vi "Save Shooting Info.vi"(1 "Turret":dbl, 2 "Pitch":dbl, 3 "RPM":dbl) -> ()   [LabVIEW 2011]
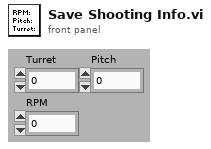
[diagram p1: front panel]
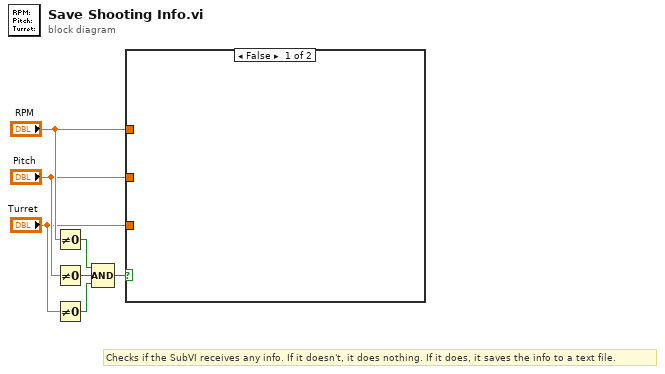
[diagram p0: block diagram]
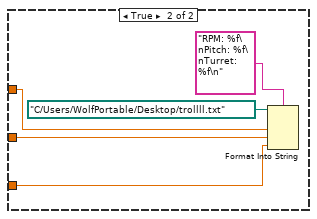
[diagram p2: hidden frame]
diagram:
  # "Checks if the SubVI receives any info. If it doesn't, it does nothing. If it does, it saves the info to a text file."
  n1 = Not Equal To 0?(x="RPM") -> (x != 0?=w7:bool)
  n2 = Not Equal To 0?(x="Pitch") -> (x != 0?=w6:bool)
  n3 = Not Equal To 0?(x="Turret") -> (x != 0?=w5:bool)
  n4 = Compound Arithmetic op=AND(w7, w6, w5) -> (w1:bool)
  n5 = case shown="False" w1 {
    tunnel: "RPM" -> [_ w10]
    tunnel: "Pitch" -> [_ w9]
    tunnel: "Turret" -> [_ w8]
    frame False {
    }
    frame True {
      n6 = Format Into String(format string="RPM: %f\nPitch: %f\nTurret: %f\n", initial string=path "C:/Users/WolfPortable/Desktop/trollll.txt" ("file path (dialog if empty)"), w10, w9, w8) -> ()  [unwired: 1 in, 2 out]
    }
  }
